vi "reset buffer.vi"(8 "error in (no error)":errorcluster, 11 "DeviceRefnum":u64) -> (0 "error out":errorcluster, 2 "function return":i32, 3 "DeviceRefnum Out":u64)   [LabVIEW 2015, in "rtlsdr.lvlib"]
doc: "Resets the streaming buffer."
uses:
  rtlsdr.lvlib
  rtlsdr/rtlsdr.dll
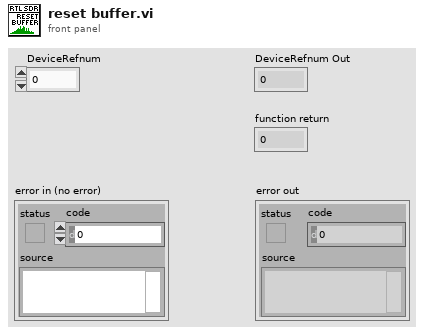
[diagram p1: front panel]
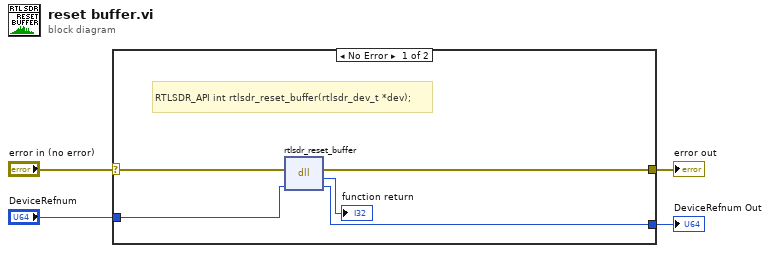
[diagram p0: block diagram]
diagram:
  n1 = case shown="No Error" "error in (no error)" {
    selector: "error in (no error)" -> [w5 w10]
    tunnel: [w8 w10] -> w4
    tunnel: "DeviceRefnum" -> [w7 w11]
    tunnel: [w6 w11] -> w2
    frame No Error {
      # "RTLSDR_API int rtlsdr_reset_buffer(rtlsdr_dev_t *dev);"
      n2 = dll-call lib="C:/Users/TheDoctor/Documents/Projects/Labview Libraries/rtlsdr/rtlsdr.*" fn="rtlsdr_reset_buffer"(error in=w5, "DeviceRefnum"=w7) -> (error out=w8:errorcluster, "return type"=→"function return":i32, "DeviceRefnum"=w6:u64)  [unwired: 2 in, 1 out]
    }
    frame Error {
    }
  }
  "error out" <- w4
  "DeviceRefnum Out" <- w2
